vi "BCU诊断标定.vi"(8 "CAN端口":u16(ring), 9 "设备索引号":u16(ring), 10 "CAN卡类型":u32(ring)=21, 11 "Myindex":dbl=1.0) -> (3 "成功":bool)   [LabVIEW 2013] (continued)
            tunnel: w101 -> [w105 _]
            tunnel: w103 -> [w104 w111]
            tunnel: w102 -> [_ w110]
            frame #0 {
              n49 = case shown="假" w105 {
                tunnel: w104 -> [w107 _]
                frame False {
                  n50 = Build Array("文件格式错误") -> (w108:string[])
                  n51 = call "表格编辑.vi"("新元素/子数组"=w108, "活动单元格:单元格背景色"=u32 16711680, "MCListbox引用句柄"=w107) -> ()  [unwired: 9 out]
                }
                frame True {
                }
              }
            }
            frame #1 {
              n52 = case shown="假" w110 {
                tunnel: w111 -> [w113 _]
                frame False {
                  n53 = Build Array("文件MD5码验证错误") -> (w114:string[])
                  n54 = call "表格编辑.vi"("新元素/子数组"=w114, "活动单元格:单元格背景色"=u32 16711680, "MCListbox引用句柄"=w113) -> ()  [unwired: 9 out]
                }
                frame True {
                }
              }
            }
          }
          n55 = call <vilib>:"Unset Busy.vi"() -> ()  [unwired: 11 in, 1 out]
        }
        frame True {
          n56 = stacked-sequence {
            seq-local: [w122 _ _ _] -> [_ w350 w444 _]
            seq-local: [w120 _ _ _] -> [_ w328 _ _]
            tunnel: w117 -> [w118 _ _ _]
            tunnel: w116 -> [w135 _ _ w471]
            frame #0 {
              w119 = string[][] []
              w132 = "总信息" ("section")
              n57 = local write "路径"(w118) -> ()
              n58 = call <vilib>:"Open Config Data.vi"("create file if necessary (T)"=FALSE, "configuration file path"=w118) -> ("error out"=w123:errorcluster, "refnum"=w122:T19)  [unwired: 7 in, 1 out]
              n59 = call <vilib>:"Get Key Names.vi"("section"=w132, "error in (no error)"=w123, "refnum"=w122) -> ("key names"=w131:string[], "refnum out"=w133:T19)  [unwired: 5 in, 2 out]
              n60 = for {
                tunnel: w133 -> [w139]
                tunnel: w132 -> [w138]
                tunnel: w131 -> [w137] mode=indexing
                tunnel: [w136] -> w128 mode=indexing
                n61 = call-poly <vilib>:"Read Key.vi"("section"=w138, "key"=w137, "refnum"=w139) -> ("value"=w136:string)  [unwired: 5 in, 3 out]
              }
              n62 = Index Array(array=w128) -> (element #1=w121:string, element #2=w126:string)  [unwired: 2 in]
              n63 = Decimal String To Number(string=w121) -> (number=w120:i32)  [unwired: 2 in, 1 out]
              n64 = Concatenate Strings("正在读取" ("字符串"), w126, "的配置文件" ("字符串")) -> (w124:string)
              n65 = Build Array(w124) -> (w129:string[])
              n66 = call "表格编辑.vi"("新元素/子数组"=w129, "活动单元格:单元格背景色"=u32 6618880, "MCListbox引用句柄"=w135) -> ()  [unwired: 9 out]
              n67 = local write "项目信息"(w119) -> ()
              n68 = local write "项目信息 2"(w119) -> ()
            }
            frame #1 {
              w310 = 20 ("长度")
              w351 = "主板" ("section")
              n69 = call <vilib>:"Get Key Names.vi"("section"=w351, "refnum"=w350) -> ("key names"=w152:string[], "refnum out"=w352:T19)  [unwired: 6 in, 2 out]
              n70 = for {
                tunnel: w352 -> [w364]
                tunnel: w351 -> [w363]
                tunnel: w152 -> [w362] mode=indexing
                tunnel: [w361] -> w151 mode=indexing
                n71 = call-poly <vilib>:"Read Key.vi"("section"=w363, "key"=w362, "refnum"=w364) -> ("value"=w361:string)  [unwired: 5 in, 3 out]
              }
              n72 = Search 1D Array(1D array=w152, element="总电压过高一级" ("元素"), start index (0)=0 ("开始索引(0)")) -> (index of element=w232:i32)
              n73 = Search 1D Array(1D array=w152, element="风机开启温度" ("元素"), start index (0)=w232) -> (index of element=w223:i32)
              n74 = Search 1D Array(1D array=w152, element="电池串联" ("元素"), start index (0)=w223) -> (index of element=w221:i32)
              n75 = Decrement(x=w232) -> (x-1=w349:i32)
              n76 = Array Subset(array=w152, index=1 ("索引"), length=w349) -> (w197:string[])
              n77 = Array Subset(array=w151, index=1 ("索引"), length=w349) -> (w194:string[])
              n78 = Delete From Array(array=w194, length=7 ("长度"), index=0 ("索引")) -> (deleted portion=w191:string[], array with subset deleted=w141:string[])
              n79 = Delete From Array(array=w197, length=7 ("长度"), index=0 ("索引")) -> (array with subset deleted=w150:string[])  [unwired: 1 out]
              n80 = Search 1D Array(1D array=w152, element="分流器型号" ("元素")) -> (index of element=w155:i32)  [unwired: 1 in]
              n81 = Index Array(array=w151, index=0 ("索引")) -> (element=w325:string)
              n82 = Decimal String To Number(string=w325) -> (number=w142:i32)  [unwired: 2 in, 1 out]
              n83 = Search 1D Array(1D array=w150, element="主板电池节数" ("元素")) -> (index of element=w316:i32)  [unwired: 1 in]
              n84 = Search 1D Array(1D array=w150, element="主板温度起始值" ("元素")) -> (index of element=w313:i32)  [unwired: 1 in]
              n85 = Search 1D Array(1D array=w150, element="第一个保险通道" ("元素")) -> (index of element=w312:i32)  [unwired: 1 in]
              n86 = Search 1D Array(1D array=w150, element="主板温度个数" ("元素")) -> (index of element=w314:i32)  [unwired: 1 in]
              n87 = Search 1D Array(1D array=w150, element="主板电压起始值" ("元素")) -> (index of element=w315:i32)  [unwired: 1 in]
              n88 = Search 1D Array(1D array=w150, element="第1通道电压个数" ("元素")) -> (index of element=w311:i32)  [unwired: 1 in]
              n89 = Index Array(array=w151, index=w155) -> (element=w154:string)
              n90 = for {
                N: 4 -> [_]
                tunnel: w191 -> [w360] mode=indexing
                tunnel: [w359] -> w340 mode=indexing
                n91 = Fract/Exp String To Number(string=w360) -> (number=w359:dbl)  [unwired: 3 in, 1 out]
              }
              n92 = Increment(x=w142) -> (x+1=w324:i32)
              n93 = Increment(x=w142) -> (x+1=w309:i32)
              n94 = Increment(x=w142) -> (x+1=w322:i32)
              n95 = Increment(x=w142) -> (x+1=w323:i32)
              n96 = global write "读配置文件全局.vi" "从板个数"(w142) -> ()
              n97 = local write "从板个数"(w142) -> ()
              n98 = Decimal String To Number(string=w154) -> (number=w153:i32)  [unwired: 2 in, 1 out]
              n99 = Index Array(array=w191, index #1=4 ("索引"), index #2=5 ("索引"), index #3=6 ("索引")) -> (element #1=w331:string, element #2=w330:string, element #3=w329:string)
              n100 = Index Array(array=w340) -> (element #1=w338:dbl, element #2=w337:dbl, element #3=w336:dbl, element #4=w335:dbl)  [unwired: 4 in]
              n101 = global write "EV05全局变量1.vi" "分流器型号"(w153) -> ()
              n102 = Array Subset(array=w141, index=w316, length=w324) -> (w308:string[])
              n103 = Array Subset(array=w141, index=w315, length=w323) -> (w306:string[])
              n104 = Array Subset(array=w141, index=w314, length=w322) -> (w305:string[])
              n105 = Array Subset(array=w141, index=w313, length=w309) -> (w304:string[])
              n106 = Array Subset(array=w141, index=w312, length=20 ("长度")) -> (w303:string[])
              n107 = Array Subset(array=w141, index=w311, length=w310) -> (w307:string[])
              n108 = Multiply(x=w142, y=2) -> (x*y=w143:i32)
              n109 = control-ref of="项目信息2"() -> (w343:refnum<vi>)
              n110 = Array Subset(array=w141, index=0 ("索引"), length=w143) -> (w140:string[])
              n111 = Insert Into Array(array=w308, new element #1=w307, new element #2=w306, new element #3=w305, new element #4=w304, new element #5=w303) -> ()  [unwired: 1 in, 1 out]
              n112 = property class="Clust (严格)"(reference=w343) -> (reference out=w341:refnum<vi>, "Value"=w342:T9)  [unwired: 1 in, 1 out]
              n113 = Multiply(x=w142, y=2) -> (x*y=w147:i32)
              n114 = Array Subset(array=w150, index=w316, length=w309) -> (w181:string[])
              n115 = Array Subset(array=w150, index=w315, length=w309) -> (w179:string[])
              n116 = Array Subset(array=w150, index=w314, length=w309) -> (w178:string[])
              n117 = Array Subset(array=w150, index=w313) -> (w177:string[])  [unwired: 1 in]
              n118 = Array Subset(array=w150, index=w312, length=w310) -> (w176:string[])
              n119 = Array Subset(array=w150, index=w311, length=w310) -> (w180:string[])
              n120 = Array Subset(array=w150, index=0 ("索引"), length=w147) -> (w146:string[])
              n121 = global write "读配置文件全局.vi" "表格输入"(w140) -> ()
              n122 = Build Array(w146, w140) -> (w302:string[][])
              n123 = Bundle(cluster=w342, "电池额定容量(A)"=w338, "使用者"=w328, "电池实际容量(A)"=w337, "车架(牌)号"=w330, "配置文件版本"=w329, "SOH(%)"=w335, "SOC(%)"=w336, "产品编号"=w331) -> (w168:T9)  [unwired: 1 in]
              n124 = Transpose 2D Array(2D array=w302) -> (transposed array=w169:string[][])
              n125 = Multiply(x=w142, y=4) -> (x*y=w173:i32)
              n126 = Insert Into Array(array=w181, new element #1=w180, new element #2=w179, new element #3=w178, new element #4=w177, new element #5=w176) -> (w175:string[])  [unwired: 1 in]
              n127 = Add(x=w173, y=44) -> (x+y=w171:i32)
              n128 = local write "项目信息"(w169) -> ()
              n129 = property class="Clust (严格)"(reference=w341, "Value"=w168) -> ()  [unwired: 1 in, 2 out]
              n130 = global write "读配置文件全局.vi" "项目信息"(w168) -> ()
              n131 = Array Subset(array=w151, index=w221, length=15 ("长度")) -> (w159:string[])
              n132 = Array Subset(array=w175, index=0 ("索引"), length=w171) -> ()  [unwired: 1 out]
              n133 = Array Subset(array=w151, index=w223, length=15 ("长度")) -> (w228:string[])
              n134 = Delete From Array(array=w159, length=4 ("长度"), index=6 ("索引")) -> (deleted portion=w215:string[], array with subset deleted=w214:string[])
              n135 = for {
                tunnel: w228 -> [w356] mode=indexing
                tunnel: [w355] -> w227 mode=indexing
                n136 = Fract/Exp String To Number(string=w356) -> (number=w355:dbl)  [unwired: 3 in, 1 out]
              }
              n137 = for {
                tunnel: w214 -> [w354] mode=indexing
                tunnel: [w353] -> w213 mode=indexing
                n138 = Fract/Exp String To Number(string=w354) -> (number=w353:dbl)  [unwired: 3 in, 1 out]
              }
              n139 = Array Subset(array=w151, index=w232, length=51 ("长度")) -> (w301:string[])
              n140 = for {
                tunnel: w301 -> [w358] mode=indexing
                tunnel: [w357] -> w300 mode=indexing
                n141 = Fract/Exp String To Number(string=w358) -> (number=w357:dbl)  [unwired: 3 in, 1 out]
              }
              n142 = Index Array(array=w213) -> (element #1=w208:dbl, element #2=w207:dbl, element #3=w206:dbl, element #4=w205:dbl, element #5=w204:dbl, element #6=w203:dbl, element #7=w202:dbl, element #8=w201:dbl, element #9=w200:dbl, element #10=w199:dbl, element #11=w198:dbl)  [unwired: 11 in]
              n143 = Delete From Array(array=w227, length=7 ("长度"), index=0 ("索引")) -> (deleted portion=w164:dbl[], array with subset deleted=w225:dbl[])
              n144 = Delete From Array(array=w300, length=17 ("长度"), index=0 ("索引")) -> (deleted portion=w161:dbl[], array with subset deleted=w297:dbl[])
              n145 = Array To Cluster(array=w164) -> (cluster=w226:T20)
              n146 = global write "读配置文件全局.vi" "加热控制参数"(w164) -> ()
              n147 = Index Array(array=w225) -> (element #1=w189:dbl, element #2=w188:dbl, element #3=w187:dbl, element #4=w186:dbl, element #5=w185:dbl, element #6=w184:dbl, element #7=w183:dbl, element #8=w182:dbl)  [unwired: 8 in]
              n148 = Delete From Array(array=w297, length=17 ("长度"), index=0 ("索引")) -> (deleted portion=w160:dbl[], array with subset deleted=w157:dbl[])
              n149 = Index Array(array=w215) -> (element #1=w212:string, element #2=w211:string, element #3=w209:string, element #4=w210:string)  [unwired: 4 in]
              n150 = local write "加热控制参数"(w226) -> ()
              n151 = global write "读配置文件全局.vi" "一级故障"(w161) -> ()
              n152 = local read "一级故障 5"() -> (w190:T12)
              n153 = control-ref of="电池信息"() -> (w219:refnum<vi>)
              n154 = global write "读配置文件全局.vi" "二级故障"(w160) -> ()
              n155 = global write "读配置文件全局.vi" "三级故障"(w157) -> ()
              n156 = Bundle(cluster=w190, "最大允许单体电压"=w189, "最大允许总电压"=w185, "最小允许单体电压"=w188, "最大允许充电电流"=w187, "最小允许充电电流"=w186, "最大允许充电温度"=w184, "最小允许充电温度"=w183, "电流步长"=w182) -> (w163:T12)
              n157 = property class="Clust (严格)"(reference=w219) -> (reference out=w220:refnum<vi>, "Value"=w218:T13)  [unwired: 1 in, 1 out]
              n158 = Bundle(cluster=w218, "电池串联"=w208, "电池并联"=w207, "累计放电总安时"=w201, "电池包额定容量"=w206, "电池包额定能量(kWh)"=w205, "电池包额定总电压"=w204, "累计充电总安时"=w202, "电池充满次数"=w199, "电池放空次数"=w200, "电池充电次数"=w198, "电池生产日期"=w209, "电池厂家"=w212, "电池类型"=w211, "电池包组号"=w210, "实际容量"=w203) -> (w158:T13)  [unwired: 2 in]
              n159 = Cluster To Array(cluster=w163) -> (array=w162:dbl[])
              n160 = local write "一级故障 5"(w163) -> ()
              n161 = global write "读配置文件全局.vi" "充电控制参数"(w162) -> ()
              n162 = Index Array(array=w161) -> (element #1=w290:dbl, element #2=w289:dbl, element #3=w288:dbl, element #4=w287:dbl, element #5=w286:dbl, element #6=w285:dbl, element #7=w284:dbl, element #8=w283:dbl, element #9=w282:dbl, element #10=w281:dbl, element #11=w280:dbl, element #12=w279:dbl, element #13=w278:dbl, element #14=w277:dbl, element #15=w276:dbl, element #16=w275:dbl, element #17=w274:dbl)  [unwired: 17 in]
              n163 = global write "读配置文件全局.vi" "电池信息"(w158) -> ()
              n164 = Index Array(array=w160) -> (element #1=w257:dbl, element #2=w258:dbl, element #3=w259:dbl, element #4=w260:dbl, element #5=w261:dbl, element #6=w262:dbl, element #7=w263:dbl, element #8=w264:dbl, element #9=w265:dbl, element #10=w266:dbl, element #11=w267:dbl, element #12=w268:dbl, element #13=w269:dbl, element #14=w270:dbl, element #15=w271:dbl, element #16=w272:dbl, element #17=w273:dbl)  [unwired: 17 in]
              n165 = Index Array(array=w157) -> (element #1=w252:dbl, element #2=w251:dbl, element #3=w250:dbl, element #4=w249:dbl, element #5=w248:dbl, element #6=w247:dbl, element #7=w246:dbl, element #8=w245:dbl, element #9=w244:dbl, element #10=w243:dbl, element #11=w242:dbl, element #12=w241:dbl, element #13=w240:dbl, element #14=w239:dbl, element #15=w238:dbl, element #16=w237:dbl, element #17=w236:dbl)  [unwired: 17 in]
              n166 = control-ref of="一级故障 3"() -> (w235:refnum<vi>)
              n167 = control-ref of="一级故障 2"() -> (w254:refnum<vi>)
              n168 = property class="Clust (严格)"(reference=w254) -> (reference out=w256:refnum<vi>, "Value"=w255:T10)  [unwired: 1 in, 1 out]
              n169 = property class="Clust (严格)"(reference=w235) -> (reference out=w234:refnum<vi>, "Value"=w253:T10)  [unwired: 1 in, 1 out]
              n170 = property class="Clust (严格)"(reference=w220, "Value"=w158) -> ()  [unwired: 1 in, 2 out]
              n171 = Bundle(cluster=w255, "总电压过高"=w257, "整组电压不均衡"=w261, "SOC过高"=w269, "单体电压过高"=w265, "总电压过低"=w258, "温度过高"=w259, "温度过低"=w260, "单组电压不均衡"=w262, "整组温度不均衡"=w263, "单组温度不均衡"=w264, "单体电压过低"=w266, "充电电流过高"=w267, "放电电流过高"=w268, "SOC过低"=w270, "内阻过大"=w271, "极柱温度过高"=w272, "SOH过低"=w273) -> (w166:T10)
              n172 = Bundle(cluster=w253, "总电压过高"=w252, "整组电压不均衡"=w248, "SOC过高"=w240, "单体电压过高"=w244, "总电压过低"=w251, "温度过高"=w250, "温度过低"=w249, "单组电压不均衡"=w247, "整组温度不均衡"=w246, "单组温度不均衡"=w245, "单体电压过低"=w243, "充电电流过高"=w242, "放电电流过高"=w241, "SOC过低"=w239, "内阻过大"=w238, "极柱温度过高"=w237, "SOH过低"=w236) -> (w165:T10)
              n173 = control-ref of="一级故障"() -> (w293:refnum<vi>)
              n174 = property class="Clust (严格)"(reference=w293) -> (reference out=w291:refnum<vi>, "Value"=w292:T10)  [unwired: 1 in, 1 out]
              n175 = Bundle(cluster=w292, "总电压过高"=w290, "整组电压不均衡"=w286, "SOC过高"=w278, "单体电压过高"=w282, "总电压过低"=w289, "温度过高"=w288, "温度过低"=w287, "单组电压不均衡"=w285, "整组温度不均衡"=w284, "单组温度不均衡"=w283, "单体电压过低"=w281, "充电电流过高"=w280, "放电电流过高"=w279, "SOC过低"=w277, "内阻过大"=w276, "极柱温度过高"=w275, "SOH过低"=w274) -> (w167:T10)
              n176 = property class="Clust (严格)"(reference=w291, "Value"=w167) -> ()  [unwired: 1 in, 2 out]
              n177 = property class="Clust (严格)"(reference=w256, "Value"=w166) -> ()  [unwired: 1 in, 2 out]
              n178 = property class="Clust (严格)"(reference=w234, "Value"=w165) -> ()  [unwired: 1 in, 2 out]
            }
            frame #2 {
              w429 = 1 ("索引")
              # "均衡计算-电压高阀值1级"
              n179 = call <vilib>:"Get Section Names.vi"("refnum"=w444) -> ("section names"=w445:string[], "refnum out"=w449:T19)  [unwired: 8 in, 1 out]
              n180 = local read "从板号"() -> (w427:u8)
              n181 = Delete From Array(array=w445, length=2 ("长度"), index=0 ("索引")) -> (array with subset deleted=w448:string[])  [unwired: 1 out]
              n182 = for {
                tunnel: w448 -> [w465] mode=indexing
                tunnel: w449 -> [w466]
                tunnel: [w458] -> w426 mode=indexing
                tunnel: [w457] -> w370
                n183 = call <vilib>:"Get Key Names.vi"("section"=w465, "refnum"=w466) -> ("key names"=w457:string[], "refnum out"=w464:T19)  [unwired: 6 in, 2 out]
                n184 = for {
                  tunnel: w457 -> [w470] mode=indexing
                  tunnel: w465 -> [w469]
                  tunnel: w464 -> [w468]
                  tunnel: [w467] -> w458 mode=indexing
                  n185 = call-poly <vilib>:"Read Key.vi"("section"=w469, "key"=w470, "refnum"=w468) -> ("value"=w467:string)  [unwired: 5 in, 3 out]
                }
                n186 = Index Array(array=w458, index=0 ("索引")) -> (element=w461:string)
                n187 = local read "输出数组"() -> (w462:string[][])
                n188 = Decimal String To Number(string=w461) -> (number=w460:i32)  [unwired: 2 in, 1 out]
                n189 = Decrement(x=w460) -> (x-1=w456:i32)
                n190 = Replace Array Subset(array=w462, new element=w458, index (col)=w456) -> (w459:string[][])  [unwired: 1 in]
                n191 = local write "输出数组"(w459) -> ()
              }
              "key names" <- w370
              n192 = Decrement(x=w427) -> (x-1=w443:u8)
              n193 = Index Array(array=w426, index (row)=w443) -> (element=w369:string[])  [unwired: 1 in]
              n194 = Search 1D Array(1D array=w370, element="风机开启温度" ("元素")) -> (index of element=w432:i32)  [unwired: 1 in]
              n195 = Search 1D Array(1D array=w370, element="电压过高一级" ("元素"), start index (0)=w432) -> (index of element=w395:i32)
              n196 = Search 1D Array(1D array=w370, element="均衡计算-电压高阀值1级" ("元素"), start index (0)=w395) -> (index of element=w393:i32)
              n197 = Array Subset(array=w369, index=w393, length=17 ("长度")) -> (w392:string[])
              n198 = Decrement(x=w432) -> (x-1=w430:i32)
              n199 = Array Subset(array=w369, index=w429, length=w430) -> (w367:string[])
              n200 = Array Subset(array=w369, index=w395, length=21 ("长度")) -> (w441:string[])
              n201 = Array Subset(array=w370, index=w429, length=w430) -> (w406:string[])
              n202 = Index Array(array=w369, index=0 ("索引")) -> (element=w401:string)
              n203 = Array Subset(array=w369, index=w432, length=7 ("长度")) -> (w435:string[])
              n204 = for {
                tunnel: w392 -> [w451] mode=indexing
                tunnel: [w450] -> w391 mode=indexing
                n205 = Fract/Exp String To Number(string=w451) -> (number=w450:dbl)  [unwired: 3 in, 1 out]
              }
              n206 = for {
                tunnel: w441 -> [w453] mode=indexing
                tunnel: [w452] -> w442 mode=indexing
                n207 = Fract/Exp String To Number(string=w453) -> (number=w452:dbl)  [unwired: 3 in, 1 out]
              }
              n208 = Decimal String To Number(string=w401) -> (number=w400:i32)  [unwired: 2 in, 1 out]
              n209 = for {
                tunnel: w435 -> [w455] mode=indexing
                tunnel: [w454] -> w403 mode=indexing
                n210 = Fract/Exp String To Number(string=w455) -> (number=w454:dbl)  [unwired: 3 in, 1 out]
              }
              n211 = global write "读配置文件全局2.vi" "从板板号"(w400) -> ()
              n212 = Delete From Array(array=w442, length=7 ("长度"), index=0 ("索引")) -> (deleted portion=w405:dbl[], array with subset deleted=w438:dbl[])
              n213 = Array To Cluster(array=w403) -> (cluster=w425:T20)
              n214 = global write "读配置文件全局2.vi" "加热控制参数"(w403) -> ()
              n215 = Delete From Array(array=w438, length=7 ("长度"), index=0 ("索引")) -> (deleted portion=w398:dbl[], array with subset deleted=w399:dbl[])
              n216 = local write "加热控制参数"(w425) -> ()
              n217 = Array To Cluster(array=w405) -> (cluster=w409:T20)
              n218 = Array To Cluster(array=w399) -> (cluster=w407:T20)
              n219 = Array To Cluster(array=w398) -> (cluster=w408:T20)
              n220 = global write "读配置文件全局2.vi" "三级故障阀值"(w399) -> ()
              n221 = global write "读配置文件全局2.vi" "一级故障阀值"(w405) -> ()
              n222 = global write "读配置文件全局2.vi" "二级故障阀值"(w398) -> ()
              n223 = local write "一级故障 6"(w409) -> ()
              n224 = local write "一级故障 8"(w407) -> ()
              n225 = local write "一级故障 7"(w408) -> ()
              n226 = Search 1D Array(1D array=w406, element="第1通道电压个数" ("元素")) -> (index of element=w417:i32)  [unwired: 1 in]
              n227 = Search 1D Array(1D array=w406, element="电压个数" ("元素")) -> ()  [unwired: 1 in, 1 out]
              n228 = Search 1D Array(1D array=w406, element="温度个数" ("元素")) -> (index of element=w419:i32)  [unwired: 1 in]
              n229 = Search 1D Array(1D array=w406, element="第一个保险通道" ("元素")) -> (index of element=w418:i32)  [unwired: 1 in]
              n230 = Array Subset(array=w367, length=2 ("长度")) -> (w414:string[])  [unwired: 1 in]
              n231 = Array Subset(array=w367, index=w419, length=2 ("长度")) -> (w412:string[])
              n232 = Array Subset(array=w367, index=w418, length=20 ("长度")) -> (w411:string[])
              n233 = Array Subset(array=w367, index=w417, length=20 ("长度")) -> (w413:string[])
              n234 = Array Subset(array=w367, length=27 ("长度")) -> (w366:string[])  [unwired: 1 in]
              n235 = Insert Into Array(array=w414, new element #1=w413, new element #2=w412, new element #3=w411) -> ()  [unwired: 1 in, 1 out]
              n236 = Build Array(string[] ["电压个数", "温度个数", "第一个保险通道", "第一个保险位置", "第二个保险通道", "第二个保险位置", "第三个保险通道", "第三个保险位置", "第四个保险通道", "第四个保险位置", "第五个保险通道", "第五个保险位置", "第六个保险通道", "第六个保险位置", "第七个保险通道", "第七个保险位置", "第八个保险通道", "第八个保险位置", "第九个保险通道", "第九个保险位置", "第十个保险通道", "第十个保险位置", "第1通道电压个数", "第2通道电压个数", "第3通道电压个数", "第4通道电压个数", "第5通道电压个数"], w366) -> (w410:string[][])
              n237 = global write "读配置文件全局2.vi" "表格"(w366) -> ()
              n238 = Index Array(array=w391) -> (element #1=w388:dbl, element #2=w387:dbl, element #3=w386:dbl, element #4=w385:dbl, element #5=w384:dbl, element #6=w383:dbl, element #7=w382:dbl, element #8=w381:dbl, element #9=w380:dbl, element #10=w379:dbl, element #11=w378:dbl, element #12=w377:dbl, element #13=w376:dbl, element #14=w375:dbl, element #15=w374:dbl, element #16=w373:dbl, element #17=w372:dbl, element #18=w371:dbl)  [unwired: 18 in]
              n239 = Transpose 2D Array(2D array=w410) -> (transposed array=w404:string[][])
              n240 = local write "项目信息 2"(w404) -> ()
              n241 = local read "均衡参数"() -> (w390:T17)
              n242 = Bundle(cluster=w390, "充电结束电压(90%)"=w381, "充电结束电压(91%)"=w380, "充电结束电压(92%)"=w379, "充电结束电压(93%)"=w378, "充电结束电压(94%)"=w377, "均衡计算-电压高阀值1级"=w388, "均衡计算-电压高阀值2级"=w387, "均衡计算-电压低阀值1级"=w386, "均衡计算-电压低阀值2级"=w385, "均衡计算-最低电压阀值"=w384, "均衡停止-最低电压阀值"=w383, "均衡计算-电压极差阀值"=w382, "充电结束电压(95%)"=w376, "充电结束电压(96%)"=w375, "充电结束电压(97%)"=w374, "充电结束电压(98%)"=w373, "充电结束电压(99%)"=w372, "充电结束电压(100%)"=w371) -> (w389:T17)
              n243 = local write "均衡参数"(w389) -> ()
            }
            frame #3 {
              n244 = call <vilib>:"Unset Busy.vi"() -> ()  [unwired: 11 in, 1 out]
              n245 = Build Array("读取完成") -> (w474:string[])
              n246 = property on="全部写入" class="Bool (严格)"("DisabledEnum"=0) -> ()  [unwired: 2 in, 2 out]
              n247 = call "表格编辑.vi"("新元素/子数组"=w474, "活动单元格:单元格背景色"=u32 6618880, "MCListbox引用句柄"=w471) -> ()  [unwired: 9 out]
            }
          }
        }
      }
    }
  }
  n248 = stacked-sequence {
    frame #0 {
    }
  }
  n249 = stacked-sequence {
    tunnel: [w488] -> w34
    frame #0 {
      w481 = 1
      w482 = string[][] []
      w501 = string[] ["", "", "", "", "", "", "", "", "", "", "", "", "", "", "", "", "", "", "", "", "", "", "", "", "", "", "", "", "", "", "", ""]
      w500 = string[][] [["", "", "", "", "", "", "", "", "", "", "", "", "", "", "", "", "", "", "", "", "", "", "", "", "", "", "", "", "", "", "", "", "", "", "", "", "", "", "", "", ""], ["", "", "", "", "", "", "", "", "", "", "", "", "", "", "", "", "", "", "", "", "", "", "", "", "", "", "", "", "", "", "", "", "", "", "", "", "", "", "", "", ""], ["", "", "", "", "", "", "", "", "", "", "", "", "", "", "", "", "", "", "", "", "", "", "", "", "", "", "", "", "", "", "", "", "", "", "", "", "", "", "", "", ""], ["", "", "", "", "", "", "", "", "", "", "", "", "", "", "", "", "", "", "", "", "", "", "", "", "", "", "", "", "", "", "", "", "", "", "", "", "", "", "", "", ""], ["", "", "", "", "", "", "", "", "", "", "", "", "", "", "", "", "", "", "", "", "", "", "", "", "", "", "", "", "", "", "", "", "", "", "", "", "", "", "", "", ""], ["", "", "", "", "", "", "", "", "", "", "", "", "", "", "", "", "", "", "", "", "", "", "", "", "", "", "", "", "", "", "", "", "", "", "", "", "", "", "", "", ""], ["", "", "", "", "", "", "", "", "", "", "", "", "", "", "", "", "", "", "", "", "", "", "", "", "", "", "", "", "", "", "", "", "", "", "", "", "", "", "", "", ""], ["", "", "", "", "", "", "", "", "", "", "", "", "", "", "", "", "", "", "", "", "", "", "", "", "", "", "", "", "", "", "", "", "", "", "", "", "", "", "", "", ""], ["", "", "", "", "", "", "", "", "", "", "", "", "", "", "", "", "", "", "", "", "", "", "", "", "", "", "", "", "", "", "", "", "", "", "", "", "", "", "", "", ""], ["", "", "", "", "", "", "", "", "", "", "", "", "", "", "", "", "", "", "", "", "", "", "", "", "", "", "", "", "", "", "", "", "", "", "", "", "", "", "", "", ""], ["", "", "", "", "", "", "", "", "", "", "", "", "", "", "", "", "", "", "", "", "", "", "", "", "", "", "", "", "", "", "", "", "", "", "", "", "", "", "", "", ""], ["", "", "", "", "", "", "", "", "", "", "", "", "", "", "", "", "", "", "", "", "", "", "", "", "", "", "", "", "", "", "", "", "", "", "", "", "", "", "", "", ""], ["", "", "", "", "", "", "", "", "", "", "", "", "", "", "", "", "", "", "", "", "", "", "", "", "", "", "", "", "", "", "", "", "", "", "", "", "", "", "", "", ""], ["", "", "", "", "", "", "", "", "", "", "", "", "", "", "", "", "", "", "", "", "", "", "", "", "", "", "", "", "", "", "", "", "", "", "", "", "", "", "", "", ""], ["", "", "", "", "", "", "", "", "", "", "", "", "", "", "", "", "", "", "", "", "", "", "", "", "", "", "", "", "", "", "", "", "", "", "", "", "", "", "", "", ""], ["", "", "", "", "", "", "", "", "", "", "", "", "", "", "", "", "", "", "", "", "", "", "", "", "", "", "", "", "", "", "", "", "", "", "", "", "", "", "", "", ""], ["", "", "", "", "", "", "", "", "", "", "", "", "", "", "", "", "", "", "", "", "", "", "", "", "", "", "", "", "", "", "", "", "", "", "", "", "", "", "", "", ""], ["", "", "", "", "", "", "", "", "", "", "", "", "", "", "", "", "", "", "", "", "", "", "", "", "", "", "", "", "", "", "", "", "", "", "", "", "", "", "", "", ""], ["", "", "", "", "", "", "", "", "", "", "", "", "", "", "", "", "", "", "", "", "", "", "", "", "", "", "", "", "", "", "", "", "", "", "", "", "", "", "", "", ""], ["", "", "", "", "", "", "", "", "", "", "", "", "", "", "", "", "", "", "", "", "", "", "", "", "", "", "", "", "", "", "", "", "", "", "", "", "", "", "", "", ""], ["", "", "", "", "", "", "", "", "", "", "", "", "", "", "", "", "", "", "", "", "", "", "", "", "", "", "", "", "", "", "", "", "", "", "", "", "", "", "", "", ""], ["", "", "", "", "", "", "", "", "", "", "", "", "", "", "", "", "", "", "", "", "", "", "", "", "", "", "", "", "", "", "", "", "", "", "", "", "", "", "", "", ""], ["", "", "", "", "", "", "", "", "", "", "", "", "", "", "", "", "", "", "", "", "", "", "", "", "", "", "", "", "", "", "", "", "", "", "", "", "", "", "", "", ""], ["", "", "", "", "", "", "", "", "", "", "", "", "", "", "", "", "", "", "", "", "", "", "", "", "", "", "", "", "", "", "", "", "", "", "", "", "", "", "", "", ""], ["", "", "", "", "", "", "", "", "", "", "", "", "", "", "", "", "", "", "", "", "", "", "", "", "", "", "", "", "", "", "", "", "", "", "", "", "", "", "", "", ""], ["", "", "", "", "", "", "", "", "", "", "", "", "", "", "", "", "", "", "", "", "", "", "", "", "", "", "", "", "", "", "", "", "", "", "", "", "", "", "", "", ""], ["", "", "", "", "", "", "", "", "", "", "", "", "", "", "", "", "", "", "", "", "", "", "", "", "", "", "", "", "", "", "", "", "", "", "", "", "", "", "", "", ""], ["", "", "", "", "", "", "", "", "", "", "", "", "", "", "", "", "", "", "", "", "", "", "", "", "", "", "", "", "", "", "", "", "", "", "", "", "", "", "", "", ""], ["", "", "", "", "", "", "", "", "", "", "", "", "", "", "", "", "", "", "", "", "", "", "", "", "", "", "", "", "", "", "", "", "", "", "", "", "", "", "", "", ""], ["", "", "", "", "", "", "", "", "", "", "", "", "", "", "", "", "", "", "", "", "", "", "", "", "", "", "", "", "", "", "", "", "", "", "", "", "", "", "", "", ""], ["", "", "", "", "", "", "", "", "", "", "", "", "", "", "", "", "", "", "", "", "", "", "", "", "", "", "", "", "", "", "", "", "", "", "", "", "", "", "", "", ""], ["", "", "", "", "", "", "", "", "", "", "", "", "", "", "", "", "", "", "", "", "", "", "", "", "", "", "", "", "", "", "", "", "", "", "", "", "", "", "", "", ""], ["", "", "", "", "", "", "", "", "", "", "", "", "", "", "", "", "", "", "", "", "", "", "", "", "", "", "", "", "", "", "", "", "", "", "", "", "", "", "", "", ""], ["", "", "", "", "", "", "", "", "", "", "", "", "", "", "", "", "", "", "", "", "", "", "", "", "", "", "", "", "", "", "", "", "", "", "", "", "", "", "", "", ""], ["", "", "", "", "", "", "", "", "", "", "", "", "", "", "", "", "", "", "", "", "", "", "", "", "", "", "", "", "", "", "", "", "", "", "", "", "", "", "", "", ""], ["", "", "", "", "", "", "", "", "", "", "", "", "", "", "", "", "", "", "", "", "", "", "", "", "", "", "", "", "", "", "", "", "", "", "", "", "", "", "", "", ""], ["", "", "", "", "", "", "", "", "", "", "", "", "", "", "", "", "", "", "", "", "", "", "", "", "", "", "", "", "", "", "", "", "", "", "", "", "", "", "", "", ""], ["", "", "", "", "", "", "", "", "", "", "", "", "", "", "", "", "", "", "", "", "", "", "", "", "", "", "", "", "", "", "", "", "", "", "", "", "", "", "", "", ""], ["", "", "", "", "", "", "", "", "", "", "", "", "", "", "", "", "", "", "", "", "", "", "", "", "", "", "", "", "", "", "", "", "", "", "", "", "", "", "", "", ""], ["", "", "", "", "", "", "", "", "", "", "", "", "", "", "", "", "", "", "", "", "", "", "", "", "", "", "", "", "", "", "", "", "", "", "", "", "", "", "", "", ""], ["", "", "", "", "", "", "", "", "", "", "", "", "", "", "", "", "", "", "", "", "", "", "", "", "", "", "", "", "", "", "", "", "", "", "", "", "", "", "", "", ""]]
      w489 = TRUE
      w484 = u32 16777215
      w480 = FALSE ("判定2")
      n250 = control-ref of="结果"() -> (w485:refnum<vi>)
      n251 = control-ref of="模块软件版本 2"() -> (w486:refnum<vi>)
      n252 = control-ref of="结果"() -> (w487:refnum<vi>)
      n253 = control-ref of="单选选项2"() -> (w504:refnum<vi>)
      n254 = control-ref of="单选选项1"() -> (w505:refnum<vi>)
      n255 = local write "key names"(string[] []) -> ()
      n256 = property on="项目信息" class="Tbl (严格)"("Disabled"=w481) -> ()  [unwired: 2 in, 2 out]
      n257 = property on="电池实际容量(A)" class="DigNum (严格)"("Disabled"=w481) -> ()  [unwired: 2 in, 2 out]
      n258 = property on="使用者" class="DigNum (严格)"("Disabled"=w481) -> ()  [unwired: 2 in, 2 out]
      n259 = property on="SOH(%)" class="DigNum (严格)"("Disabled"=w481) -> ()  [unwired: 2 in, 2 out]
      n260 = property on="电池额定容量(A)" class="DigNum (严格)"("Disabled"=w481) -> ()  [unwired: 2 in, 2 out]
      n261 = local write "主从选择"(enum32{"主板", "从板"}."主板" ("主从选择")) -> ()
      n262 = property on="SOC(%)" class="DigNum (严格)"("Disabled"=w481) -> ()  [unwired: 2 in, 2 out]
      n263 = local write "等级 2"(T21."从板信息" ("等级 2")) -> ()
      n264 = local write "主板2"(T8."项目信息" ("主从板")) -> ()
      n265 = property class="MCListbox (严格)"(reference=w487, "ItemNames"=w482) -> ()  [unwired: 1 in, 2 out]
      n266 = property class="MCListbox (严格)"(reference=w486, "ItemNames"=w482) -> ()  [unwired: 1 in, 2 out]
      n267 = property class="MCListbox (严格)"(reference=w485, "ItemNames"=w482) -> ()  [unwired: 1 in, 2 out]
      n268 = property class="Bool (严格)"(reference=w504, "BoolText.TextColor"=u32 87470) -> ()  [unwired: 1 in, 2 out]
      n269 = property class="Bool (严格)"(reference=w505, "BoolText.TextColor"=w484) -> ()  [unwired: 1 in, 2 out]
      n270 = property on="从板号" class="DigNum (严格)"("NumText.BGColor"=w484) -> ()  [unwired: 2 in, 2 out]
      n271 = local write "主从板"(enum32{"单选选项2", "单选选项1"}."单选选项1" ("主从板")) -> ()
      n272 = property on="项目信息2" class="Clust (严格)"("DisabledEnum"=w481) -> ()  [unwired: 2 in, 2 out]
      n273 = property on="系统时钟" class="Str"("Disabled"=w481) -> ()  [unwired: 2 in, 2 out]
      n274 = property on="配置文件版本" class="Str"("Disabled"=w481) -> ()  [unwired: 2 in, 2 out]
      n275 = property on="车架(牌)号" class="Str"("Disabled"=w481) -> ()  [unwired: 2 in, 2 out]
      n276 = property on="产品编号" class="Str"("Disabled"=w481) -> ()  [unwired: 2 in, 2 out]
      n277 = local write "判定3"(w489) -> ()
      n278 = local write "清BUFF"(w489) -> ()
      n279 = local write "1"(w489) -> ()
      n280 = property on="从板个数" class="DigNum (严格)"("Visible"=w489) -> ()  [unwired: 2 in, 2 out]
      n281 = property on="从板个数" class="DigNum (严格)"("NumText.BGColor"=u32 16448250) -> ()  [unwired: 2 in, 2 out]
      n282 = Not(x=w489) -> (.not. x?=w508:bool)
      n283 = local write "布尔"(w489) -> ()
      n284 = property on="主板选项" class="Tree (严格)"("Visible"=w489) -> ()  [unwired: 2 in, 2 out]
      n285 = property on="全部写入" class="Bool (严格)"("DisabledEnum"=2) -> ()  [unwired: 2 in, 2 out]
      n286 = property on="从板选项" class="Tree (严格)"("Visible"=w508) -> ()  [unwired: 2 in, 2 out]
      n287 = property on="当前从板板号" class="DigNum (严格)"("Visible"=w508) -> ()  [unwired: 2 in, 2 out]
      n288 = control-ref of="结果"() -> (w495:refnum<vi>)
      n289 = control-ref of="结果"() -> (w492:refnum<vi>)
      n290 = local write "强制停止版本读取"(w480) -> ()
      n291 = local write "强制终止读写标记"(w480) -> ()
      n292 = control-ref of="项目信息"() -> (w493:refnum<vi>)
      n293 = local write "判定2"(w480) -> ()
      n294 = local write "停止"(w480) -> ()
      n295 = local write "控制1"(w480) -> ()
      n296 = local write "消除"(w480) -> ()
      n297 = global write "EV05全局变量1.vi" "授权功能"(w480) -> ()
      n298 = local write "继电器超时处理"(w480) -> ()
      n299 = local write "1 6"(w480) -> ()
      n300 = local write "1 7"(w480) -> ()
      n301 = local write "1 8"(w480) -> ()
      n302 = local write "1 9"(w480) -> ()
      n303 = local write "1 10"(w480) -> ()
      n304 = local write "1 2"(w480) -> ()
      n305 = local write "1 3"(w480) -> ()
      n306 = local write "1 4"(w480) -> ()
      n307 = local write "1 5"(w480) -> ()
      n308 = local write "1 11"(w480) -> ()
      n309 = for {
        N: 150 -> [_]
        tunnel: w495 -> [w536]
        i -> [w534]
        n310 = Bundle(w534, 0) -> (w532:cluster{i32, i32})  [unwired: 1 out]
        n311 = property class="MCListbox (严格)"(reference=w536, "ActiveCell"=w532, "CellBG"=u32 16448250) -> ()  [unwired: 1 in, 2 out]
      }
      n312 = for {
        N: 150 -> [_]
        tunnel: w493 -> [w531]
        i -> [w530]
        n313 = Bundle(w530, 0) -> (w528:cluster{i32, i32})  [unwired: 1 out]
        n314 = property class="Tbl (严格)"(reference=w531, "Active Cell"=w528, "Cell BG Color"=u32 16448250) -> ()  [unwired: 1 in, 2 out]
      }
      n315 = for {
        N: 150 -> [_]
        tunnel: w492 -> [w541]
        i -> [w539]
        n316 = Bundle(w539, 0) -> (w537:cluster{i32, i32})  [unwired: 1 out]
        n317 = property class="MCListbox (严格)"(reference=w541, "ActiveCell"=w537, "CellBG"=u32 16448250) -> ()  [unwired: 1 in, 2 out]
      }
      n318 = stacked-sequence {
        tunnel: [_ _ w515] -> w488
        frame #0 {
          w509 = u32 21 items=["PCI5121"=1, "PCI9810"=2, "USBCAN1"=3, "USBCAN2"=4, "PCI9820"=5, "PCI5110"=7, "CANLite(mini)"=8, "ISA9620"=9, "ISA5420"=10, "PC104CAN"=11, "DNP9810"=13, "PCI9840B"=14, "PC104C2"=15, "PCI9820I"=16, "pec9920"=18, "USBCAN_E_U"=20, "USBCAN_2E_U"=21] ("CAN卡类型")
          n319 = local write "CAN卡类型"(w509) -> ()
        }
        frame #1 {
          n320 = disable-structure shown="禁用" {
            frame Disabled {
              n321 = local read "设备索引号"() -> (w511:u16)
              n322 = local read "CAN卡类型"() -> (w510:u32)
              n323 = local read "CAN端口"() -> (w512:u16)
              n324 = dll-call lib="PTH1abs FBluewave New EnergySVN_WorkAutoTest_TestStandtrunkAutoTest_TestStandDriverZlgCanBHN01è¯»ååæ°data\nkerneldlls\nusbcan.dll" fn="VCI_ClearBuffer"("DeviceType"=w510, "DeviceInd"=w511, "CANInd"=w512) -> (error out=w513:errorcluster)  [unwired: 4 in, 4 out]
              n325 = call <vilib>:"Clear Errors.vi"("error in (no error)"=w513) -> ()  [unwired: 6 in, 1 out]
            }
            frame Enabled {
            }
          }
        }
        frame #2 {
          w522 = u8 0 items=["Normal", "Listen Only"] ("工作方式")
          w521 = u8 1 items=["Dual Filter", "Single Filter"] ("滤波方式")
          n326 = local read "设备索引号"() -> (w517:u16)
          n327 = local read "CAN卡类型"() -> (w516:u32)
          n328 = local read "CAN端口"() -> (w518:u16)
          n329 = call "CAN_Init-8.6.vi"("CAN卡类型"=w516, "设备索引号"=w517, "CAN端口"=w518, "操作类型"=enum16{"初始化CAN", "关闭CAN"}."初始化CAN", "滤波方式"=w521, "Accept Code"=u32 3221225472, "簇"=T23 {"打开CAN"=TRUE, "初始化CAN"=TRUE, "开始CAN"=TRUE, "重启"=FALSE, "关闭CAN"=FALSE}, "Mask Code"=u32 1073741823 ("Accept Code"), "工作方式"=w522, "是否滤波"=TRUE, "滤波选择"=T22 {"fiter_mode"=1, "fiter_endid"=402653184, "fiter_startid"=419430399}) -> ("CAN 操作结果"=→"CAN":bool, "error out"=w515:errorcluster)  [unwired: 3 in, 4 out]
        }
      }
      n330 = local write "加热继电器(从)"(w480) -> ()
      n331 = local write "风机继电器(从)"(w480) -> ()
      n332 = local write "DO1"(w480) -> ()
      n333 = local write "DO2"(w480) -> ()
      n334 = local write "DO1 2"(w480) -> ()
      n335 = local write "正级继电器"(w480) -> ()
      n336 = local write "负级继电器"(w480) -> ()
      n337 = local write "加热继电器"(w480) -> ()
      n338 = local write "充电继电器"(w480) -> ()
      n339 = local write "风机继电器"(w480) -> ()
      n340 = local write "预充电继电器"(w480) -> ()
      n341 = property on="保存版本信息" class="Bool (严格)"("Visible"=w480) -> ()  [unwired: 2 in, 2 out]
      n342 = property on="单个读取" class="Bool (严格)"("Visible"=w480) -> ()  [unwired: 2 in, 2 out]
      n343 = property on="单个写入" class="Bool (严格)"("Visible"=w480) -> ()  [unwired: 2 in, 2 out]
      n344 = local write "正级继电器 12"(w480) -> ()
      n345 = local write "正级继电器 2"(w480) -> ()
      n346 = local write "正级继电器 3"(w480) -> ()
      n347 = local write "正级继电器 4"(w480) -> ()
      n348 = local write "正级继电器 5"(w480) -> ()
      n349 = local write "正级继电器 6"(w480) -> ()
      n350 = local write "正级继电器 7"(w480) -> ()
      n351 = local write "正级继电器 8"(w480) -> ()
      n352 = local write "正级继电器 9"(w480) -> ()
      n353 = local write "正级继电器 10"(w480) -> ()
      n354 = local write "正级继电器 11"(w480) -> ()
      n355 = property on="从板号" class="DigNum (严格)"("Visible"=w480) -> ()  [unwired: 2 in, 2 out]
      "电池故障" <- w482
      "模块版本值" <- w500
      "硬件版本" <- w501
      "模块版本名称" <- w500
      "平台软件版本" <- w501
      "项目软件版本" <- w501
      "模块个数" <- u8[] [0, 0, 0, 0, 0, 0, 0, 0, 0, 0, 0, 0, 0, 0, 0, 0, 0, 0, 0, 0, 0, 0, 0, 0, 0, 0, 0, 0, 0, 0, 0, 0] ("模块个数")
    }
  }
  n356 = stacked-sequence {
    tunnel: [w542] -> w37
    frame #0 {
      n357 = call <vilib>:"Set Busy.vi"() -> ()  [unwired: 10 in, 2 out]
      n358 = disable-structure shown="禁用" {
        frame Disabled {
          n359 = control-ref of="主板选项"() -> (w661:refnum<vi>)
          n360 = stacked-sequence {
            tunnel: w661 -> [w663 w821 w859]
            frame #0 {
              # "加热和充电控制参数"
              n361 = global read "功能码全局.vi" "主板控制类信息10"() -> (w673:bool[])
              n362 = Index Array(array=w673) -> (element #5=w667:bool, element #6=w665:bool, element #7=w666:bool, element #8=w664:bool)  [unwired: 8 in, 4 out]
              n363 = Not Or(1:w666, 2:w667) -> (0:w672:bool)
              n364 = Not Or(1:w664, 2:w665) -> (0:w670:bool)
              n365 = for {
                N: 8 -> [_]
                tunnel: w663 -> [w793]
                tunnel: w672 -> [w789]
                tunnel: [w788] -> w671
                i -> [w791]
                n366 = Add(x=w791, y=69) -> (x+y=w792:i32)
                n367 = property class="Tree (严格)"(reference=w793, "Active Item Row Number"=w792, "Disabled?"=w789) -> (error out=w788:errorcluster)  [unwired: 1 in, 1 out]
              }
              n368 = for {
                N: 9 -> [_]
                tunnel: w663 -> [w787]
                tunnel: w670 -> [w783]
                tunnel: w671 -> [w782]
                tunnel: [w781] -> w662
                i -> [w785]
                n369 = Add(x=w785, y=77) -> (x+y=w786:i32)
                n370 = property class="Tree (严格)"(reference=w787, error in=w782, "Active Item Row Number"=w786, "Disabled?"=w783) -> (error out=w781:errorcluster)  [unwired: 1 out]
              }
              n371 = stacked-sequence {
                tunnel: w663 -> [w693 _ _]
                tunnel: w662 -> [w692 _ _]
                frame #0 {
                  # "电池信息"
                  n372 = global read "功能码全局.vi" "主板版本号11"() -> (w694:bool[])
                  n373 = global read "功能码全局.vi" "主板项目信息4"() -> (w676:bool[])
                  n374 = Index Array(array=w694) -> (element #1=w690:bool, element #2=w689:bool, element #3=w683:bool, element #4=w677:bool, element #6=w682:bool, element #7=w681:bool, element #8=w680:bool)  [unwired: 8 in, 1 out]
                  n375 = Index Array(array=w676, index=4 ("索引")) -> (element=w674:bool)
                  n376 = Or(x=w683, y=w677) -> (x .or. y?=w678:bool)
                  n377 = Not(x=w681) -> (.not. x?=w685:bool)
                  n378 = Not(x=w680) -> (.not. x?=w684:bool)
                  n379 = Not(x=w682) -> (.not. x?=w686:bool)
                  n380 = property on="硬件版本号" class="Str"("Visible"=w683) -> ()  [unwired: 2 in, 2 out]
                  n381 = property on="读硬件版本号" class="Bool (严格)"("Visible"=w683) -> ()  [unwired: 2 in, 2 out]
                  n382 = property on="项目软件版本号" class="Str"("Visible"=w683) -> ()  [unwired: 2 in, 2 out]
                  n383 = property on="项目软本读取" class="Bool (严格)"("Visible"=w683) -> ()  [unwired: 2 in, 2 out]
                  n384 = property on="继电器屏1 2" class="TabCtl (严格)"("Visible"=w686) -> ()  [unwired: 2 in, 2 out]
                  n385 = property on="均衡屏" class="TabCtl (严格)"("Visible"=w684) -> ()  [unwired: 2 in, 2 out]
                  n386 = property on="继电器屏1 2" class="TabCtl (严格)"("Visible"=w686) -> ()  [unwired: 2 in, 2 out]
                  n387 = property on="DO屏" class="TabCtl (严格)"("Visible"=w685) -> ()  [unwired: 2 in, 2 out]
                  n388 = Compound Arithmetic op=OR(w682, w681, w680) -> (w679:bool)
                  n389 = Not Or(1:w689, 2:w690) -> (0:w688:bool)
                  n390 = stacked-sequence {
                    tunnel: w679 -> [_ w699 _]
                    tunnel: w678 -> [_ _ w703]
                    tunnel: w674 -> [w695 _ _]
                    frame #0 {
                      n391 = case shown="真" w695 {
                        frame False {
                        }
                        frame True {
                          n392 = local write "主界面选项"(enum32{"单选选项1", "单选选项2", "单选选项2 2", "单选选项2 3"}."单选选项2 3" ("主界面选项")) -> ()
                          n393 = local write "面板选择"(T7."高压板校正" ("面板选择")) -> ()
                        }
                      }
                      n394 = control-ref of="单选选项2 3"() -> (w696:refnum<vi>)
                      n395 = property class="Bool (严格)"(reference=w696, "Visible"=w695) -> ()  [unwired: 1 in, 2 out]
                    }
                    frame #1 {
                      n396 = control-ref of="单选选项2 2"() -> (w700:refnum<vi>)
                      n397 = case shown="真" w699 {
                        frame False {
                        }
                        frame True {
                          n398 = local write "主界面选项"(enum32{"单选选项1", "单选选项2", "单选选项2 2", "单选选项2 3"}."单选选项2 2" ("主界面选项")) -> ()
                          n399 = local write "面板选择"(enum32{"读写参数", "版本读取", "其它诊断"}."其它诊断" ("选项卡控件 2")) -> ()
                        }
                      }
                      n400 = property class="Bool (严格)"(reference=w700, "Visible"=w699) -> ()  [unwired: 1 in, 2 out]
                    }
                    frame #2 {
                      n401 = control-ref of="单选选项2"() -> (w704:refnum<vi>)
                      n402 = case shown="真" w703 {
                        frame False {
                        }
                        frame True {
                          n403 = local write "主界面选项"(enum32{"单选选项1", "单选选项2", "单选选项2 2", "单选选项2 3"}."单选选项2" ("主界面选项")) -> ()
                          n404 = local write "面板选择"(enum32{"读写参数", "版本读取", "其它诊断"}."版本读取" ("选项卡控件 2")) -> ()
                        }
                      }
                      n405 = property class="Bool (严格)"(reference=w704, "Visible"=w703) -> ()  [unwired: 1 in, 2 out]
                    }
                  }
                  n406 = for {
                    N: 5 -> [_]
                    tunnel: w693 -> [w713]
                    tunnel: w688 -> [w709]
                    tunnel: w692 -> [w708]
                    tunnel: [w707] -> w691
                    i -> [w711]
                    n407 = Add(x=w711, y=86) -> (x+y=w712:i32)
                    n408 = property class="Tree (严格)"(reference=w713, error in=w708, "Active Item Row Number"=w712, "Disabled?"=w709) -> (error out=w707:errorcluster)  [unwired: 1 out]
                  }
                  n409 = property on="模块软件版本 2" class="MCListbox (严格)"("Visible"=w677) -> ()  [unwired: 2 in, 2 out]
                  n410 = property on="模块软件版本" class="Enum (严格)"("Visible"=w677) -> ()  [unwired: 2 in, 2 out]
                  n411 = property on="平台软件版本号" class="Str"("Visible"=w677) -> ()  [unwired: 2 in, 2 out]
                  n412 = property on="模块版本读取" class="Bool (严格)"("Visible"=w677) -> ()  [unwired: 2 in, 2 out]
                  n413 = property on="平台软件版本读取" class="Bool (严格)"("Visible"=w677) -> ()  [unwired: 2 in, 2 out]
                  n414 = call <vilib>:"Clear Errors.vi"("error in (no error)"=w691) -> ()  [unwired: 6 in, 1 out]
                }
                frame #1 {
                  n415 = global read "功能码全局.vi" "主板项目信息7"() -> (w753:bool[])
                  n416 = global read "功能码全局.vi" "主板控制类信息10"() -> (w749:bool[])
                  n417 = global read "功能码全局.vi" "主板故障阀值9"() -> (w752:bool[])
                  n418 = global read "功能码全局.vi" "主板项目信息4"() -> (w731:bool[])
                  n419 = global read "功能码全局.vi" "主板项目信息5"() -> (w740:bool[])
                  n420 = global read "功能码全局.vi" "主板项目信息6"() -> (w730:bool[])
                  n421 = global read "功能码全局.vi" "主板版本号11"() -> (w739:bool[])
                  n422 = Delete From Array(array=w730, length=1 ("长度"), index=0 ("索引")) -> (deleted portion=w741:bool[], array with subset deleted=w757:bool[])
                  n423 = Index Array(array=w731, index #1=5 ("索引"), index #2=6 ("索引"), index #3=7 ("索引")) -> (element #1=w742:bool, element #2=w758:bool, element #3=w714:bool)
                  n424 = Index Array(array=w739) -> (element #1=w746:bool, element #2=w762:bool)  [unwired: 2 in]
                  n425 = Array Subset(array=w752, index=2 ("索引"), length=3 ("长度")) -> (w744:bool[])
                  n426 = Delete From Array(array=w753, length=3 ("索引"), index=2 ("长度")) -> (deleted portion=w743:bool[], array with subset deleted=w759:bool[])
                  n427 = Array Subset(array=w749, index=4 ("索引"), length=2 ("长度")) -> (w745:bool[])
                  n428 = global read "功能码全局.vi" "18"() -> (w722:bool[])
                  n429 = global read "功能码全局.vi" "16"() -> (w723:bool[])
                  n430 = Insert Into Array(array=w740, new element #1=w741, new element #2=w742, new element #3=w743, new element #4=w744, new element #5=w745, new element #6=w746) -> (w763:bool[])  [unwired: 1 in]
                  n431 = Array Subset(array=w749, index=6 ("索引"), length=2 ("长度")) -> (w761:bool[])
                  n432 = Array Subset(array=w752, index=5 ("索引"), length=3 ("长度")) -> (w760:bool[])
                  n433 = And Array Elements(Boolean array=w763) -> (logical AND=w728:bool)
                  n434 = Array Subset(array=w722, index=0 ("索引"), length=8 ("长度")) -> (w720:bool[])
                  n435 = Array Subset(array=w723, index=4 ("索引"), length=4 ("长度")) -> (w719:bool[])
                  n436 = Or Array Elements(Boolean array=w763) -> (logical OR=w715:bool)
                  n437 = Insert Into Array(array=w757, new element #1=w758, new element #2=w759, new element #3=w760, new element #4=w761, new element #5=w762) -> (w764:bool[])  [unwired: 1 in]
                  n438 = property on="全部读取" class="Bool (严格)"("Visible"=w728) -> ()  [unwired: 2 in, 2 out]
                  n439 = global read "功能码全局.vi" "15"() -> (w721:bool[])
                  n440 = And Array Elements(Boolean array=w764) -> (logical AND=w729:bool)
                  n441 = property on="全部写入" class="Bool (严格)"("Visible"=w729) -> ()  [unwired: 2 in, 2 out]
                  n442 = Or Array Elements(Boolean array=w764) -> (logical OR=w765:bool)
                  n443 = Insert Into Array(array=w721, new element #1=w720, new element #2=w719) -> (w718:bool[])  [unwired: 1 in]
                  n444 = Or Array Elements(Boolean array=w718) -> (logical OR=w717:bool)
                  n445 = Compound Arithmetic op=OR(w714, w715, w765, w717) -> (w766:bool)
                  n446 = case shown="真" w766 {
                    frame False {
                    }
                    frame True {
                      n447 = local write "主界面选项"(enum32{"单选选项1", "单选选项2", "单选选项2 2", "单选选项2 3"}."单选选项1" ("主界面选项")) -> ()
                      n448 = local write "面板选择"(enum32{"读写参数", "版本读取", "其它诊断"}."读写参数" ("选项卡控件 2")) -> ()
                    }
                  }
                  n449 = property on="单选选项1" class="Bool (严格)"("Visible"=w766) -> ()  [unwired: 2 in, 2 out]
                }
                frame #2 {
                  n450 = control-ref of="单选选项2 2"() -> (w773:refnum<vi>)
                  n451 = control-ref of="单选选项2 3"() -> (w769:refnum<vi>)
                  n452 = control-ref of="单选选项2"() -> (w775:refnum<vi>)
                  n453 = control-ref of="单选选项1"() -> (w774:refnum<vi>)
                  n454 = local read "主界面选项"() -> (w778:enum32{"单选选项1", "单选选项2", "单选选项2 2", "单选选项2 3"})
                  n455 = Build Array(w774, w775, w773, w769) -> (w772:refnum<vi>[])
                  n456 = Delete From Array(array=w772, index=w778) -> (deleted portion=w776:refnum<vi>, array with subset deleted=w777:refnum<vi>[])  [unwired: 1 in]
                  n457 = property class="Bool (严格)"(reference=w776, "BoolText.TextColor"=u32 87470) -> ()  [unwired: 1 in, 2 out]
                  n458 = for {
                    tunnel: u32 16777215 -> [w780]
                    tunnel: w777 -> [w779] mode=indexing
                    n459 = property class="Bool (严格)"(reference=w779, "BoolText.TextColor"=w780) -> ()  [unwired: 1 in, 2 out]
                  }
                }
              }
            }
            frame #1 {
              # "项目信息"
              # "SOC"
              # "SOH"
              # "电池额定实际容量"
              # "车牌号"
              # "产品编号"
              # "电压个数"
              # "通道电压数"
              # "温度个数"
              # "电压起始值"
              # "温度起始值"
              # "配置文件版本"
              # "系统时钟"
              # "校正时钟"
              n460 = global read "功能码全局.vi" "主板项目信息5"() -> (w854:bool[])
              n461 = global read "功能码全局.vi" "主板项目信息6"() -> (w853:bool[])
              n462 = global read "功能码全局.vi" "主板项目信息7"() -> (w830:bool[])
              n463 = global read "功能码全局.vi" "主板项目信息4"() -> (w801:bool[])
              n464 = Index Array(array=w854) -> (element #1=w851:bool, element #2=w848:bool, element #3=w845:bool, element #4=w842:bool, element #5=w838:bool, element #6=w836:bool, element #7=w833:bool, element #8=w829:bool)  [unwired: 8 in]
              n465 = Index Array(array=w853) -> (element #1=w826:bool, element #2=w850:bool, element #3=w847:bool, element #4=w844:bool, element #5=w841:bool, element #6=w837:bool, element #7=w835:bool, element #8=w832:bool)  [unwired: 8 in]
              n466 = Index Array(array=w830) -> (element #1=w828:bool, element #2=w825:bool, element #3=w823:bool, element #4=w818:bool, element #5=w815:bool, element #6=w822:bool, element #7=w816:bool, element #8=w814:bool)  [unwired: 8 in]
              n467 = Index Array(array=w801) -> (element #6=w797:bool, element #7=w796:bool, element #8=w800:bool)  [unwired: 8 in, 5 out]
              n468 = Not(x=w800) -> (.not. x?=w799:bool)
              n469 = Not Or(1:w796, 2:w797) -> (0:w795:bool)
              n470 = Not Or(1:w850, 2:w851) -> (0:w813:bool)
              n471 = Not Or(1:w847, 2:w848) -> (0:w812:bool)
              n472 = Not Or(1:w844, 2:w845) -> (0:w811:bool)
              n473 = Not Or(1:w841, 2:w842) -> (0:w810:bool)
              n474 = Not Or(1:w837, 2:w838) -> (0:w809:bool)
              n475 = Not Or(1:w835, 2:w836) -> (0:w808:bool)
              n476 = Not Or(1:w832, 2:w833) -> (0:w807:bool)
              n477 = Not Or(1:w828, 2:w829) -> (0:w806:bool)
              n478 = Not Or(1:w822, 2:w823) -> (0:w804:bool)
              n479 = Not Or(1:w814, 2:w815) -> (0:w802:bool)
              n480 = Not Or(1:w816, 2:w818) -> (0:w803:bool)
              n481 = Not Or(1:w825, 2:w826) -> (0:w805:bool)
              n482 = Compound Arithmetic op=OR(w799, w813, w812, w811, w810, w809, w808, w807, w806, w805, w804, w803, w802) -> (w794:bool)
              "项目信息结果" <- w794
